vi "whole_setup_control_FPGA_v1229.vi"() -> ()   [LabVIEW 2021]
uses:
  <vilib>/rvi/Emulation/niFpgaSctlEmulationGetInTimedLoop.vi
  <vilib>/rvi/Emulation/niFpgaProcessEmulError.vi
  <vilib>/rvi/Emulation/niFpgaGetClockAttributes.vi
  <vilib>/rvi/Emulation/niFpgaEmulationReportErrorSimple.vi
  <vilib>/rvi/Emulation/niFpgaCriticalErrorInLSC.vi
  <vilib>/rvi/interface/RandomDataEmulation/niFpgaRandomDataHandleErrors.vi
  <vilib>/rvi/Memory/Memory_Emulation/nirvimemoryFastEmulation.vi
  <vilib>/rvi/Memory/Memory_Emulation/nirvimemoryEmulation.vi
  <vilib>/rvi/Emulation/niFpgaEmulationIsFPGAContextNoSignature.vi
  <vilib>/rvi/DataTransferAndStorage/Container/Common/niFpgaContainerGetUniqueNameForEmu.vi
  <vilib>/rvi/errors/nirviReportUnexpectedCaseInternalError (U32).vi
  <vilib>/rvi/eio/common/nirviEmuTemplateMethod_errors.vi
  <vilib>/rvi/DataTransferAndStorage/Container/XNode/niFpgaContainer.xnode
  <vilib>/rvi/interface/RandomDataEmulation/nirviRandomDataFpgaReadWriteTemplate.vi
  <vilib>/eio/EIOMethodNode/EIOMethodNode.xnode
  <vilib>/eio/EIONode/EIONode.xnode
  <vilib>/rvi/FXPMathLib/FxpMul/XNode/nifxpmath_Multiplier.xnode
  <vilib>/rvi/FXPMathLib/FxpAdd/XNode/nifxpmath_Add.xnode
  <vilib>/rvi/FXPMathLib/sim/FxpSim.dll
panel:
  in  "laser ON":bool
  out "Cycle tick spent":u32
  in  "camera trigger ON":bool
  out "FIFO Full? 2":bool
  in  "FPGA loop case":u32 caption="output loop ticks"
  in  "trigger debug?":bool
  in  "DO 4 delay":i32
  in  "DO 3 delay":i32
  in  "camera trigger delay (loops)":i32
  in  "laser delay (loops)":i32
  in  "laser exposure (loops)":i32
  in  "3F0 freq X":i32=3
  in  "2F0 freq X":i32=5
  out "ticks spent update":u32
  out "Loop ticks spent":u32
  in  "Galvo1 offset":fxp<+/-,32,16>
  in  "Galvo1 mag":fxp<+/-,32,16>
  in  "G1 corr amplitude":fxp<+/-,32,16>
  in  "Piezo offset":fxp<+/-,32,16>
  in  "Piezo mag":fxp<+/-,32,16>
  in  "3F0 amplitude":fxp<+/-,32,16>
  in  "2F0 amplitude":fxp<+/-,32,16>
  in  "Galvo1 delay":i32
  in  "Galvo1 corr delay":i32
  in  "stop output":bool
  in  "2F0 phase relative to F0":i32
  in  "3F0 phase relative to F0":i32
  in  "output loop ticks":u32
  in  "output data #":i32
  in  "start output":bool
  in  "array length":i16
  in  "FPGA start to read FIFO":bool
  in  "data row #":i32
  out "Data transfer finished":bool=TRUE
  out "FPGA finish read row":bool
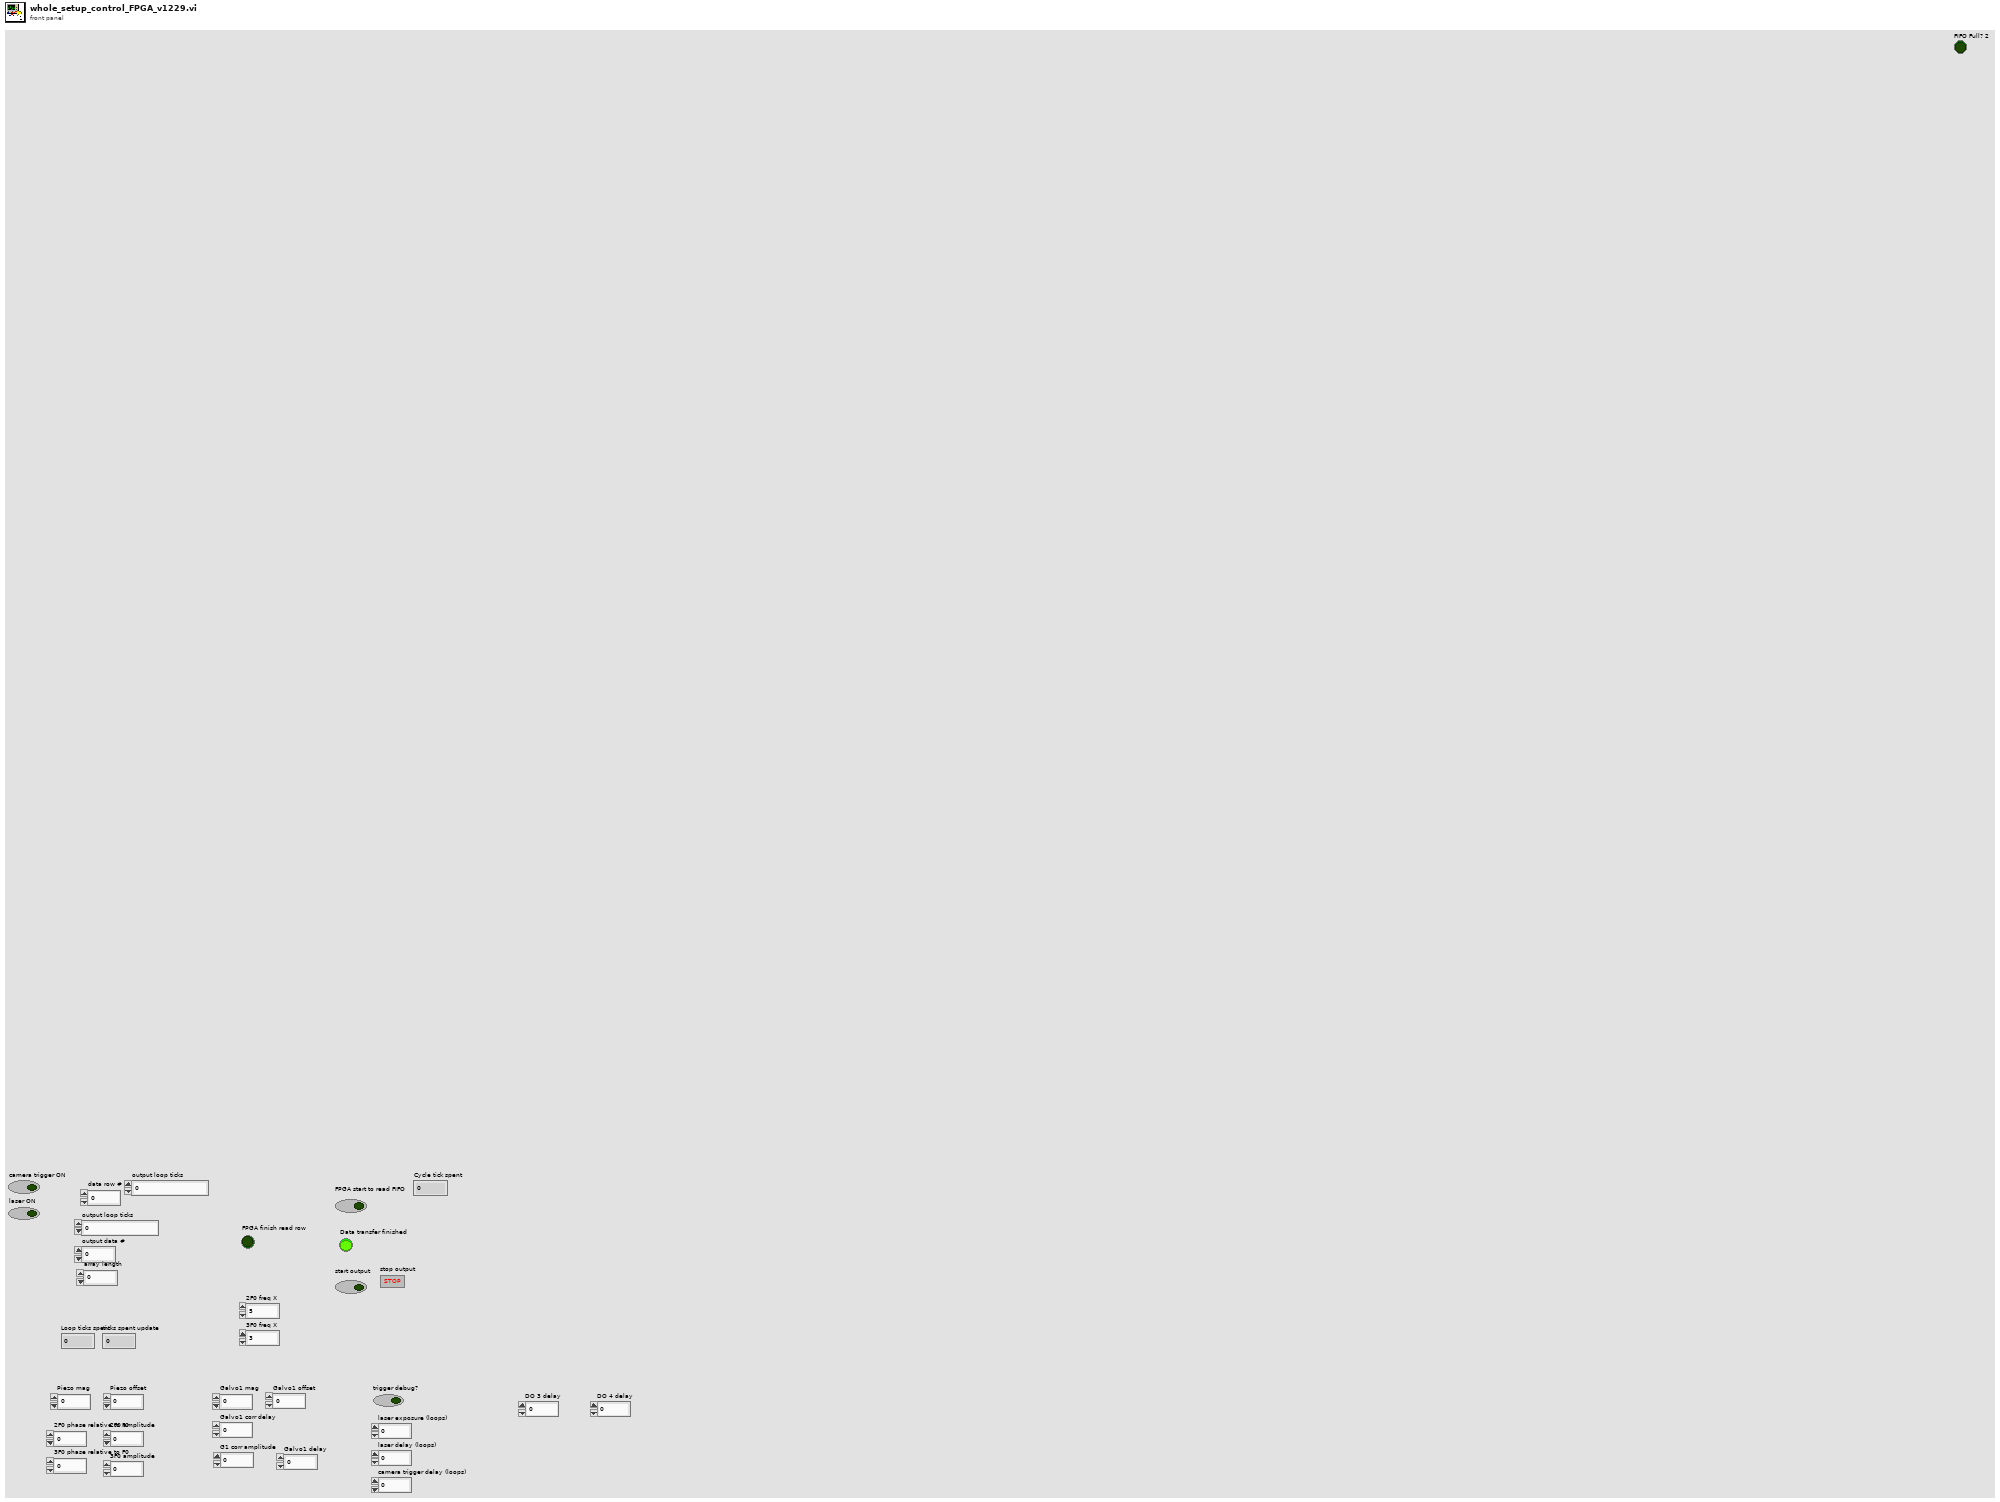
[diagram p1: front panel]
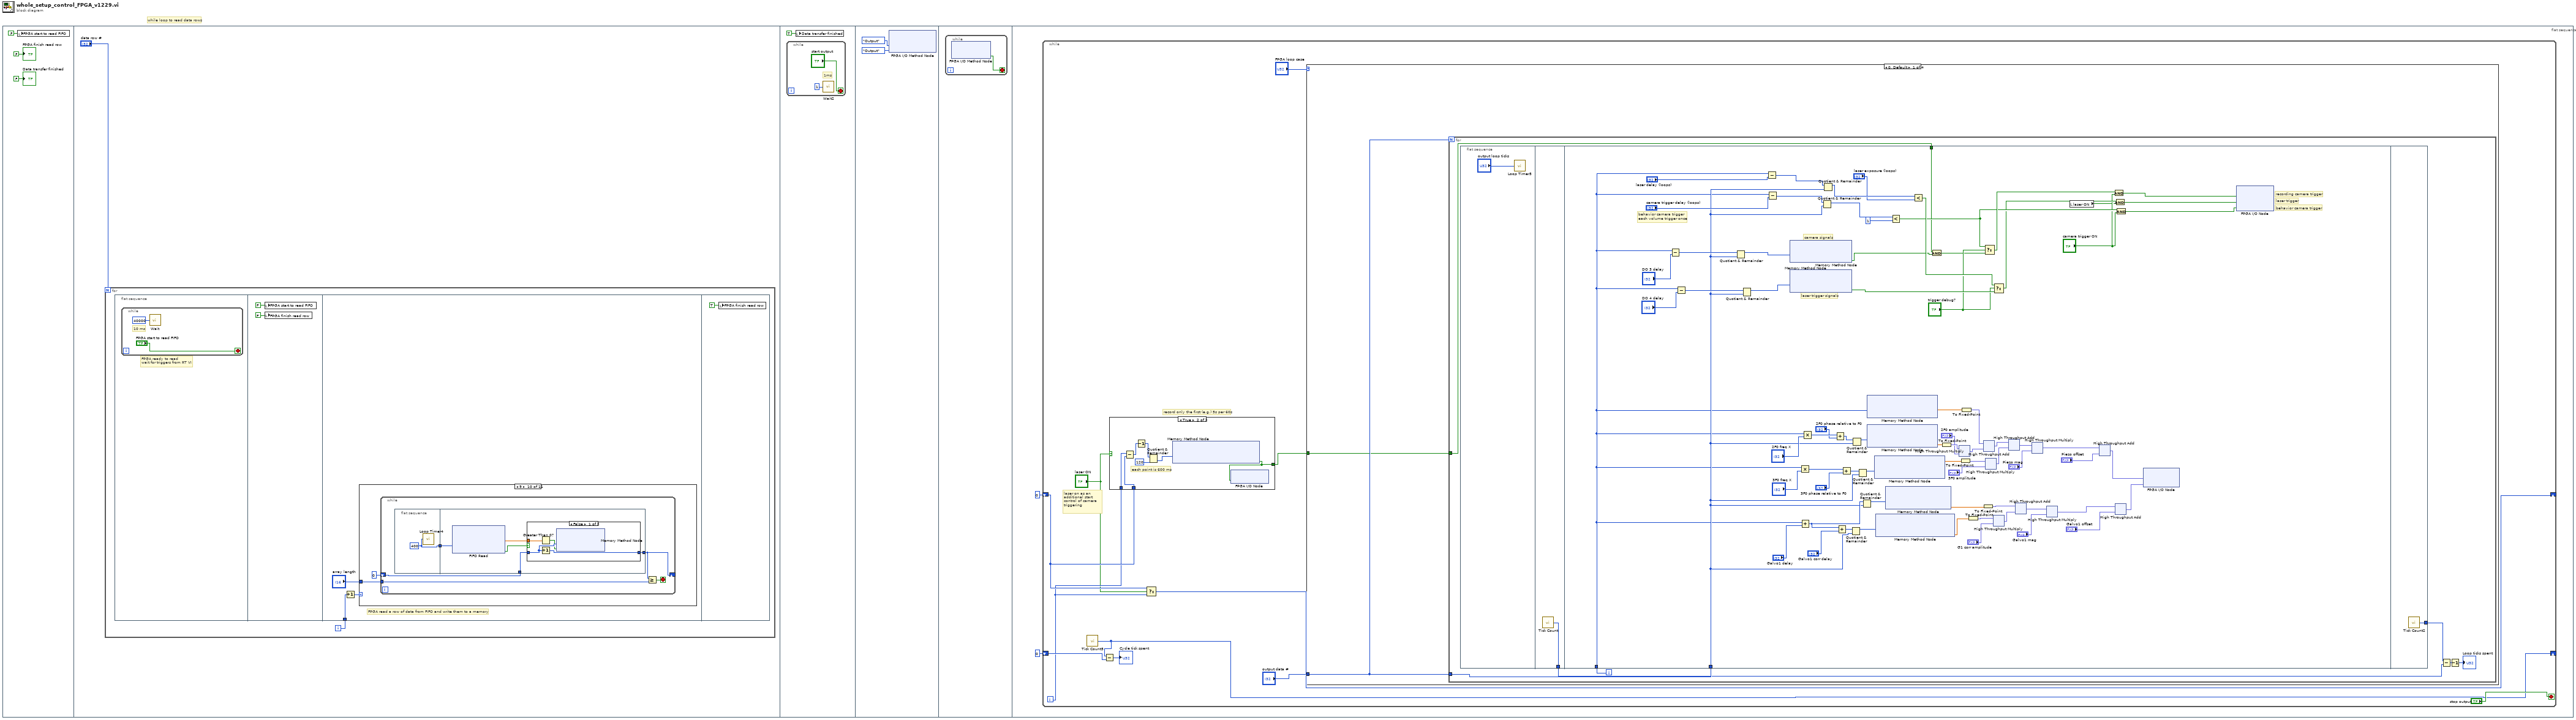
[diagram p0: block diagram]
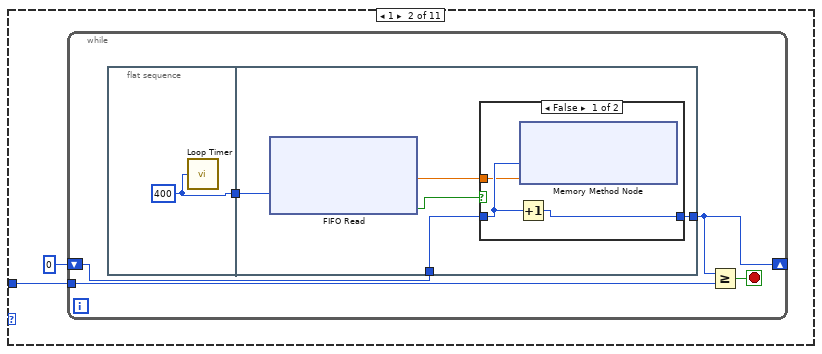
[diagram p3: hidden frame]
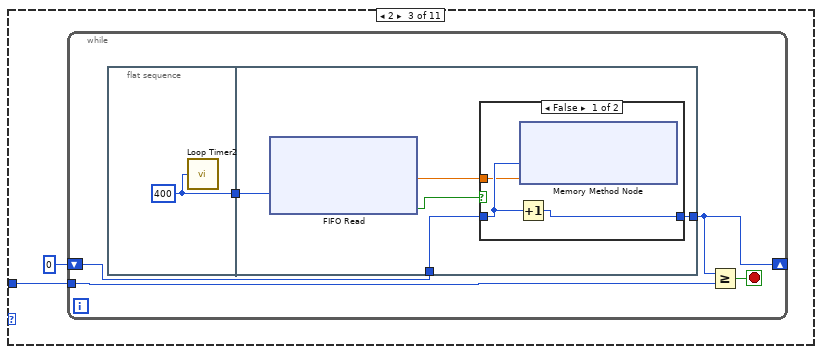
[diagram p5: hidden frame]
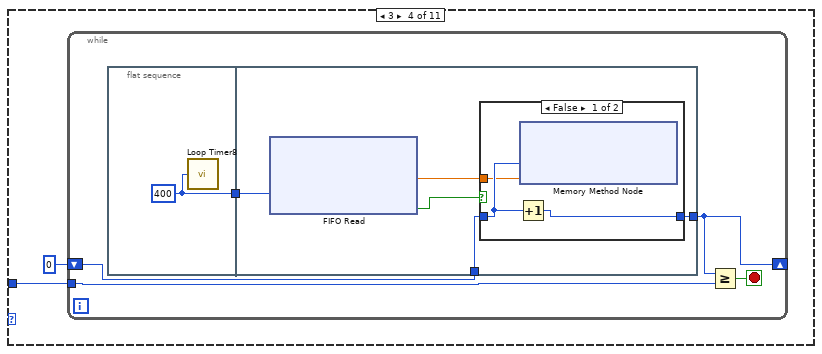
[diagram p7: hidden frame]
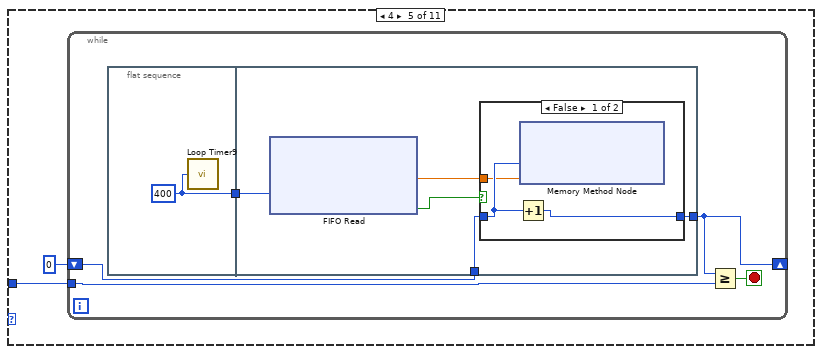
[diagram p9: hidden frame]
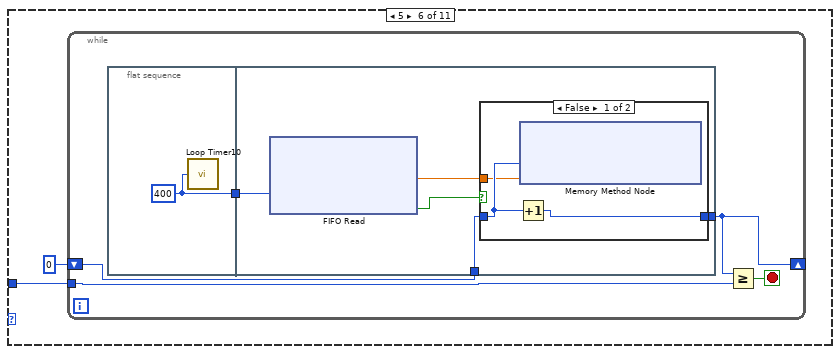
[diagram p11: hidden frame]
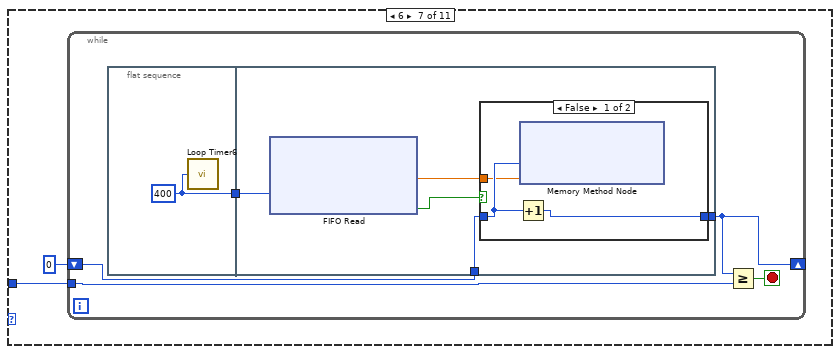
[diagram p13: hidden frame]
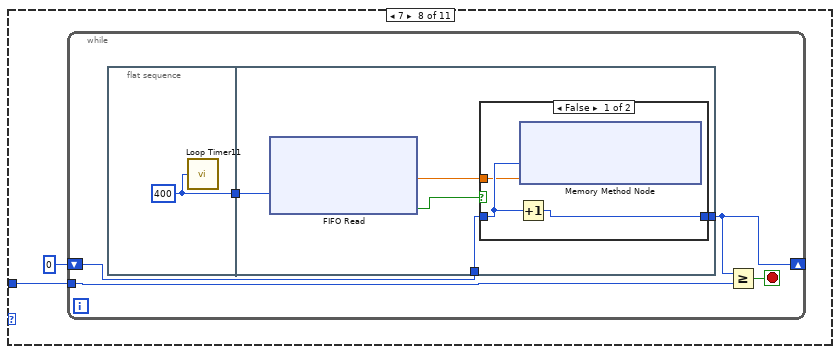
[diagram p15: hidden frame]
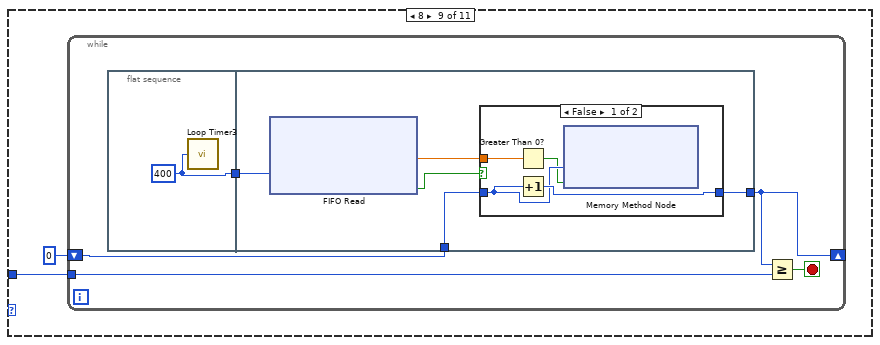
[diagram p17: hidden frame]
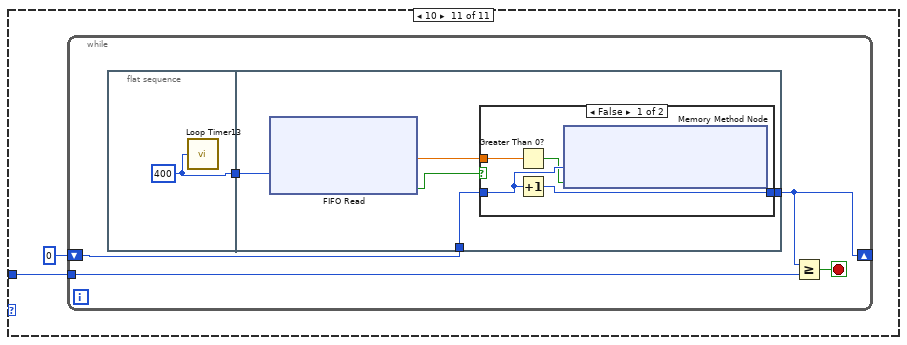
[diagram p20: hidden frame]
diagram:
  # "while loop to read data rows"
  n1 = flat-sequence {
    frame #0 {
      n2 = local write "FPGA start to read FIFO"(FALSE ("FPGA ready to read")) -> ()
      "Data transfer finished" <- FALSE ("Data transfer finished")
      "FPGA finish read row" <- FALSE ("FPGA ready to read")
    }
    frame #1 {
      n3 = for {
        N: "data row #" -> [_]
        i -> [w5]
        n4 = flat-sequence {
          tunnel: w5 -> [w10]
          frame #0 {
            # "FPGA ready to read\nwait for triggers from RT VI"
            n5 = while {
              stop <- "FPGA start to read FIFO" stop-if-true
              # "10 ms"
              n6 = call "Wait"("Count(Ticks)"=u32 40000) -> ()  [unwired: 1 out]
            }
          }
          frame #1 {
            n7 = local write "FPGA start to read FIFO"(FALSE ("FPGA ready to read")) -> ()
            n8 = local write "FPGA finish read row"(FALSE ("FPGA finish read row")) -> ()
          }
          frame #2 {
            # "FPGA read a row of data from FIFO and write them to a memory"
            n9 = Increment(x=w10) -> (x+1=w11:i32)
            n10 = case shown="9" w11 {
              tunnel: "array length" -> [_ w13 w30 w47 w64 w81 w98 w115 w132 w150 w168]
              frame 0, Default {
              }
              frame 1 {
                n11 = while {
                  shift-right: [w15] -> _
                  shift-left: i16 0 -> [w19]
                  tunnel: w13 -> [w16]
                  stop <- w17 stop-if-true
                  n12 = flat-sequence {
                    tunnel: [w20] -> w18
                    tunnel: w19 -> [w24]
                    tunnel: [w23] -> w15
                    tunnel: w18 -> [w21]
                    frame #0 {
                      w20 = u32 400 ("Count(Ticks)")
                      n13 = call "Loop Timer"("Count(Ticks)"=w20) -> ()  [unwired: 1 out]
                    }
                    frame #1 {
                      n14 = xnode ("FIFO Read")("Timeout"=w21) -> ("Element"=w25:sgl, "Timed Out?"=w22:bool)  [unwired: 1 in, 1 out]
                      n15 = case shown="False" w22 {
                        tunnel: w25 -> [w26 _]
                        tunnel: w24 -> [w27 w29]
                        tunnel: [w28 w29] -> w23
                        frame False {
                          n16 = Increment(x=w27) -> (x+1=w28:i16)
                          n17 = xnode ("Memory Method Node")("Address"=w27, "Data"=w26) -> ()  [unwired: 1 in, 1 out]
                        }
                        frame True {
                        }
                      }
                    }
                  }
                  n18 = Greater Or Equal?(x=w15, y=w16) -> (x >= y?=w17:bool)
                }
              }
              frame 2 {
                n19 = while {
                  shift-right: [w32] -> _
                  shift-left: i16 0 -> [w36]
                  tunnel: w30 -> [w33]
                  stop <- w34 stop-if-true
                  n20 = flat-sequence {
                    tunnel: [w37] -> w35
                    tunnel: w36 -> [w41]
                    tunnel: [w40] -> w32
                    tunnel: w35 -> [w38]
                    frame #0 {
                      w37 = u32 400 ("Count(Ticks)")
                      n21 = call "Loop Timer2"("Count(Ticks)"=w37) -> ()  [unwired: 1 out]
                    }
                    frame #1 {
                      n22 = xnode ("FIFO Read")("Timeout"=w38) -> ("Element"=w42:sgl, "Timed Out?"=w39:bool)  [unwired: 1 in, 1 out]
                      n23 = case shown="False" w39 {
                        tunnel: w42 -> [w43 _]
                        tunnel: w41 -> [w44 w46]
                        tunnel: [w45 w46] -> w40
                        frame False {
                          n24 = Increment(x=w44) -> (x+1=w45:i16)
                          n25 = xnode ("Memory Method Node")("Address"=w44, "Data"=w43) -> ()  [unwired: 1 in, 1 out]
                        }
                        frame True {
                        }
                      }
                    }
                  }
                  n26 = Greater Or Equal?(x=w32, y=w33) -> (x >= y?=w34:bool)
                }
              }
              frame 3 {
                n27 = while {
                  shift-right: [w49] -> _
                  shift-left: i16 0 -> [w53]
                  tunnel: w47 -> [w50]
                  stop <- w51 stop-if-true
                  n28 = flat-sequence {
                    tunnel: [w54] -> w52
                    tunnel: w53 -> [w58]
                    tunnel: [w57] -> w49
                    tunnel: w52 -> [w55]
                    frame #0 {
                      w54 = u32 400 ("Count(Ticks)")
                      n29 = call "Loop Timer8"("Count(Ticks)"=w54) -> ()  [unwired: 1 out]
                    }
                    frame #1 {
                      n30 = xnode ("FIFO Read")("Timeout"=w55) -> ("Element"=w59:sgl, "Timed Out?"=w56:bool)  [unwired: 1 in, 1 out]
                      n31 = case shown="False" w56 {
                        tunnel: w59 -> [w60 _]
                        tunnel: w58 -> [w61 w63]
                        tunnel: [w62 w63] -> w57
                        frame False {
                          n32 = Increment(x=w61) -> (x+1=w62:i16)
                          n33 = xnode ("Memory Method Node")("Address"=w61, "Data"=w60) -> ()  [unwired: 1 in, 1 out]
                        }
                        frame True {
                        }
                      }
                    }
                  }
                  n34 = Greater Or Equal?(x=w49, y=w50) -> (x >= y?=w51:bool)
                }
              }
              frame 4 {
                n35 = while {
                  shift-right: [w66] -> _
                  shift-left: i16 0 -> [w70]
                  tunnel: w64 -> [w67]
                  stop <- w68 stop-if-true
                  n36 = flat-sequence {
                    tunnel: [w71] -> w69
                    tunnel: w70 -> [w75]
                    tunnel: [w74] -> w66
                    tunnel: w69 -> [w72]
                    frame #0 {
                      w71 = u32 400 ("Count(Ticks)")
                      n37 = call "Loop Timer9"("Count(Ticks)"=w71) -> ()  [unwired: 1 out]
                    }
                    frame #1 {
                      n38 = xnode ("FIFO Read")("Timeout"=w72) -> ("Element"=w76:sgl, "Timed Out?"=w73:bool)  [unwired: 1 in, 1 out]
                      n39 = case shown="False" w73 {
                        tunnel: w76 -> [w77 _]
                        tunnel: w75 -> [w78 w80]
                        tunnel: [w79 w80] -> w74
                        frame False {
                          n40 = Increment(x=w78) -> (x+1=w79:i16)
                          n41 = xnode ("Memory Method Node")("Address"=w78, "Data"=w77) -> ()  [unwired: 1 in, 1 out]
                        }
                        frame True {
                        }
                      }
                    }
                  }
                  n42 = Greater Or Equal?(x=w66, y=w67) -> (x >= y?=w68:bool)
                }
              }
              frame 5 {
                n43 = while {
                  shift-right: [w83] -> _
                  shift-left: i16 0 -> [w87]
                  tunnel: w81 -> [w84]
                  stop <- w85 stop-if-true
                  n44 = flat-sequence {
                    tunnel: [w88] -> w86
                    tunnel: w87 -> [w92]
                    tunnel: [w91] -> w83
                    tunnel: w86 -> [w89]
                    frame #0 {
                      w88 = u32 400 ("Count(Ticks)")
                      n45 = call "Loop Timer10"("Count(Ticks)"=w88) -> ()  [unwired: 1 out]
                    }
                    frame #1 {
                      n46 = xnode ("FIFO Read")("Timeout"=w89) -> ("Element"=w93:sgl, "Timed Out?"=w90:bool)  [unwired: 1 in, 1 out]
                      n47 = case shown="False" w90 {
                        tunnel: w93 -> [w94 _]
                        tunnel: w92 -> [w95 w97]
                        tunnel: [w96 w97] -> w91
                        frame False {
                          n48 = Increment(x=w95) -> (x+1=w96:i16)
                          n49 = xnode ("Memory Method Node")("Address"=w95, "Data"=w94) -> ()  [unwired: 1 in, 1 out]
                        }
                        frame True {
                        }
                      }
                    }
                  }
                  n50 = Greater Or Equal?(x=w83, y=w84) -> (x >= y?=w85:bool)
                }
              }
              frame 6 {
                n51 = while {
                  shift-right: [w100] -> _
                  shift-left: i16 0 -> [w104]
                  tunnel: w98 -> [w101]
                  stop <- w102 stop-if-true
                  n52 = flat-sequence {
                    tunnel: [w105] -> w103
                    tunnel: w104 -> [w109]
                    tunnel: [w108] -> w100
                    tunnel: w103 -> [w106]
                    frame #0 {
                      w105 = u32 400 ("Count(Ticks)")
                      n53 = call "Loop Timer6"("Count(Ticks)"=w105) -> ()  [unwired: 1 out]
                    }
                    frame #1 {
                      n54 = xnode ("FIFO Read")("Timeout"=w106) -> ("Element"=w110:sgl, "Timed Out?"=w107:bool)  [unwired: 1 in, 1 out]
                      n55 = case shown="False" w107 {
                        tunnel: w110 -> [w111 _]
                        tunnel: w109 -> [w112 w114]
                        tunnel: [w113 w114] -> w108
                        frame False {
                          n56 = Increment(x=w112) -> (x+1=w113:i16)
                          n57 = xnode ("Memory Method Node")("Address"=w112, "Data"=w111) -> ()  [unwired: 1 in, 1 out]
                        }
                        frame True {
                        }
                      }
                    }
                  }
                  n58 = Greater Or Equal?(x=w100, y=w101) -> (x >= y?=w102:bool)
                }
              }
              frame 7 {
                n59 = while {
                  shift-right: [w117] -> _
                  shift-left: i16 0 -> [w121]
                  tunnel: w115 -> [w118]
                  stop <- w119 stop-if-true
                  n60 = flat-sequence {
                    tunnel: [w122] -> w120
                    tunnel: w121 -> [w126]
                    tunnel: [w125] -> w117
                    tunnel: w120 -> [w123]
                    frame #0 {
                      w122 = u32 400 ("Count(Ticks)")
                      n61 = call "Loop Timer11"("Count(Ticks)"=w122) -> ()  [unwired: 1 out]
                    }
                    frame #1 {
                      n62 = xnode ("FIFO Read")("Timeout"=w123) -> ("Element"=w127:sgl, "Timed Out?"=w124:bool)  [unwired: 1 in, 1 out]
                      n63 = case shown="False" w124 {
                        tunnel: w127 -> [w128 _]
                        tunnel: w126 -> [w129 w131]
                        tunnel: [w130 w131] -> w125
                        frame False {
                          n64 = Increment(x=w129) -> (x+1=w130:i16)
                          n65 = xnode ("Memory Method Node")("Address"=w129, "Data"=w128) -> ()  [unwired: 1 in, 1 out]
                        }
                        frame True {
                        }
                      }
                    }
                  }
                  n66 = Greater Or Equal?(x=w117, y=w118) -> (x >= y?=w119:bool)
                }
              }
              frame 8 {
                n67 = while {
                  shift-right: [w134] -> _
                  shift-left: i16 0 -> [w138]
                  tunnel: w132 -> [w135]
                  stop <- w136 stop-if-true
                  n68 = flat-sequence {
                    tunnel: [w139] -> w137
                    tunnel: w138 -> [w143]
                    tunnel: [w142] -> w134
                    tunnel: w137 -> [w140]
                    frame #0 {
                      w139 = u32 400 ("Count(Ticks)")
                      n69 = call "Loop Timer3"("Count(Ticks)"=w139) -> ()  [unwired: 1 out]
                    }
                    frame #1 {
                      n70 = xnode ("FIFO Read")("Timeout"=w140) -> ("Element"=w144:sgl, "Timed Out?"=w141:bool)  [unwired: 1 in, 1 out]
                      n71 = case shown="False" w141 {
                        tunnel: w144 -> [w146 _]
                        tunnel: w143 -> [w147 w149]
                        tunnel: [w148 w149] -> w142
                        frame False {
                          n72 = Greater Than 0?(x=w146) -> (x > 0?=w145:bool)
                          n73 = Increment(x=w147) -> (x+1=w148:i16)
                          n74 = xnode ("Memory Method Node")("Address"=w147, "Data"=w145) -> ()  [unwired: 1 in, 1 out]
                        }
                        frame True {
                        }
                      }
                    }
                  }
                  n75 = Greater Or Equal?(x=w134, y=w135) -> (x >= y?=w136:bool)
                }
              }
              frame 9 {
                n76 = while {
                  shift-right: [w152] -> _
                  shift-left: i16 0 -> [w156]
                  tunnel: w150 -> [w153]
                  stop <- w154 stop-if-true
                  n77 = flat-sequence {
                    tunnel: [w157] -> w155
                    tunnel: w156 -> [w161]
                    tunnel: [w160] -> w152
                    tunnel: w155 -> [w158]
                    frame #0 {
                      w157 = u32 400 ("Count(Ticks)")
                      n78 = call "Loop Timer4"("Count(Ticks)"=w157) -> ()  [unwired: 1 out]
                    }
                    frame #1 {
                      n79 = xnode ("FIFO Read")("Timeout"=w158) -> ("Element"=w162:sgl, "Timed Out?"=w159:bool)  [unwired: 1 in, 1 out]
                      n80 = case shown="False" w159 {
                        tunnel: w162 -> [w164 _]
                        tunnel: w161 -> [w165 w167]
                        tunnel: [w166 w167] -> w160
                        frame False {
                          n81 = Greater Than 0?(x=w164) -> (x > 0?=w163:bool)
                          n82 = Increment(x=w165) -> (x+1=w166:i16)
                          n83 = xnode ("Memory Method Node")("Address"=w165, "Data"=w163) -> ()  [unwired: 1 in, 1 out]
                        }
                        frame True {
                        }
                      }
                    }
                  }
                  n84 = Greater Or Equal?(x=w152, y=w153) -> (x >= y?=w154:bool)
                }
              }
              frame 10 {
                n85 = while {
                  shift-right: [w170] -> _
                  shift-left: i16 0 -> [w174]
                  tunnel: w168 -> [w171]
                  stop <- w172 stop-if-true
                  n86 = flat-sequence {
                    tunnel: [w175] -> w173
                    tunnel: w174 -> [w179]
                    tunnel: [w178] -> w170
                    tunnel: w173 -> [w176]
                    frame #0 {
                      w175 = u32 400 ("Count(Ticks)")
                      n87 = call "Loop Timer13"("Count(Ticks)"=w175) -> ()  [unwired: 1 out]
                    }
                    frame #1 {
                      n88 = xnode ("FIFO Read")("Timeout"=w176) -> ("Element"=w180:sgl, "Timed Out?"=w177:bool)  [unwired: 1 in, 1 out]
                      n89 = case shown="False" w177 {
                        tunnel: w180 -> [w182 _]
                        tunnel: w179 -> [w183 w185]
                        tunnel: [w184 w185] -> w178
                        frame False {
                          n90 = Greater Than 0?(x=w182) -> (x > 0?=w181:bool)
                          n91 = Increment(x=w183) -> (x+1=w184:i16)
                          n92 = xnode ("Memory Method Node")("Address"=w183, "Data"=w181) -> ()  [unwired: 1 in, 1 out]
                        }
                        frame True {
                        }
                      }
                    }
                  }
                  n93 = Greater Or Equal?(x=w170, y=w171) -> (x >= y?=w172:bool)
                }
              }
            }
          }
          frame #3 {
            n94 = local write "FPGA finish read row"(TRUE ("FPGA finish read row")) -> ()
          }
        }
      }
    }
    frame #2 {
      n95 = while {
        stop <- "start output" stop-if-true
        # "1ms"
        n96 = call "Wait2"("Count(mSec)"=u32 1) -> ()  [unwired: 1 out]
      }
      n97 = local write "Data transfer finished"(TRUE ("Data transfer finished")) -> ()
    }
    frame #3 {
      n98 = xnode "FPGA I/O Method Node"("DIO 7:4"=enum8{"No Change", "Input", "Output"}."Output", "DIO 3:0"=enum8{"No Change", "Input", "Output"}."Output") -> ()  [unwired: 1 in, 1 out]
    }
    frame #4 {
      n99 = while {
        stop <- w192 stop-if-true
        n100 = xnode "FPGA I/O Method Node"() -> ("Ready"=w192:bool)  [unwired: 2 in, 2 out]
      }
    }
    frame #5 {
      n101 = while {
        shift-right: [w202] -> _
        shift-left: u32 0 ("Tick Count(Ticks)") -> [w201]
        shift-right: [w199] -> _
        shift-left: 0 -> [w198]
        i -> [w197]
        stop <- "stop output" stop-if-true
        # "record only the first (e.g.) 5s per 60s"
        # "laser on as an additional start control of camera triggering"
        n102 = call "Tick Count5"() -> ("Tick Count(Ticks)"=w202:u32)
        n103 = Subtract(x=w202, y=w201) -> (x-y=→"Cycle tick spent":u32)
        n104 = case shown="True" "laser ON" {
          tunnel: w198 -> [_ w213]
          tunnel: w197 -> [_ w212]
          tunnel: [w206 w207] -> w195
          frame False {
            w206 = FALSE ("Mod1/DIO3")
            n105 = xnode "FPGA I/O Node"("Mod1/DIO3"=w206) -> ()  [unwired: 1 in, 1 out]
          }
          frame True {
            # "each point is 600 ms"
            n106 = Subtract(x=w212, y=w213) -> (x-y=w209:i32)
            n107 = Decrement(x=w209) -> (x-1=w208:i32)
            n108 = Quotient & Remainder(x=w208, y=120) -> (floor(x/y)=w211:i32)  [unwired: 1 out]
            n109 = xnode ("Memory Method Node")("Address"=w211) -> ("Data"=w207:bool)  [unwired: 1 in, 1 out]
            n110 = xnode "FPGA I/O Node"("Mod1/DIO3"=w207) -> ()  [unwired: 1 in, 1 out]
          }
        }
        n111 = Select(t=w198, s="laser ON", f=w197) -> (s? t:f=w199:i32)
        n112 = case shown="0, Default" "FPGA loop case" {
          tunnel: "output data #" -> [w215 w300 w326 _]
          tunnel: w195 -> [w214 _ _ _]
          frame 0, Default {
            n113 = for {
              N: w215 -> [_]
              tunnel: w215 -> [w221]
              tunnel: w214 -> [w216]
              i -> [w222]
              n114 = flat-sequence {
                tunnel: [w224] -> w218
                tunnel: w222 -> [w237]
                tunnel: w221 -> [w238]
                tunnel: w216 -> [w229]
                tunnel: [w298] -> w217
                frame #0 {
                  n115 = call "Loop Timer5"("Count(Ticks)"="output loop ticks") -> ()  [unwired: 1 out]
                }
                frame #1 {
                  n116 = call "Tick Count"() -> ("Tick Count(Ticks)"=w224:u32)
                }
                frame #2 {
                  # "recording camera trigger"
                  # "laser trigger"
                  # "behavior camera trigger"
                  # "behavior camera trigger\neach volume trigger once"
                  # "laser trigger signals"
                  # "camera signals"
                  n117 = Subtract(x=w237, y="DO 3 delay") -> (x-y=w248:i32)
                  n118 = Subtract(x=w237, y="DO 4 delay") -> (x-y=w245:i32)
                  n119 = Quotient & Remainder(x=w248, y=w238) -> (x-y*floor(x/y)=w247:i32)  [unwired: 1 out]
                  n120 = Quotient & Remainder(x=w245, y=w238) -> (x-y*floor(x/y)=w243:i32)  [unwired: 1 out]
                  n121 = Subtract(x=w237, y="laser delay (loops)") -> (x-y=w252:i32)
                  n122 = Subtract(x=w237, y="camera trigger delay (loops)") -> (x-y=w250:i32)
                  n123 = xnode ("Memory Method Node")("Address"=w247) -> ("Data"=w228:bool)  [unwired: 1 in, 1 out]
                  n124 = xnode ("Memory Method Node")("Address"=w243) -> ("Data"=w242:bool)  [unwired: 1 in, 1 out]
                  n125 = Multiply(x=w237, y="3F0 freq X") -> (x*y=w297:i32)
                  n126 = Add(x=w237, y="Galvo1 delay") -> (x+y=w258:i32)
                  n127 = Multiply(x=w237, y="2F0 freq X") -> (x*y=w293:i32)
                  n128 = Quotient & Remainder(x=w250, y=w238) -> (x-y*floor(x/y)=w225:i32)  [unwired: 1 out]
                  n129 = Quotient & Remainder(x=w252, y=w238) -> (x-y*floor(x/y)=w254:i32)  [unwired: 1 out]
                  n130 = Add(x=w293, y="2F0 phase relative to F0") -> (x+y=w296:i32)
                  n131 = Add(x=w258, y="Galvo1 corr delay") -> (x+y=w286:i32)
                  n132 = Add(x=w297, y="3F0 phase relative to F0") -> (x+y=w290:i32)
                  n133 = Quotient & Remainder(x=w286, y=w238) -> (x-y*floor(x/y)=w288:i32)  [unwired: 1 out]
                  n134 = Quotient & Remainder(x=w296, y=w238) -> (x-y*floor(x/y)=w295:i32)  [unwired: 1 out]
                  n135 = Quotient & Remainder(x=w290, y=w238) -> (x-y*floor(x/y)=w289:i32)  [unwired: 1 out]
                  n136 = Quotient & Remainder(x=w258, y=w238) -> (x-y*floor(x/y)=w256:i32)  [unwired: 1 out]
                  n137 = xnode ("Memory Method Node")("Address"=w237) -> ("Data"=w284:sgl)  [unwired: 1 in, 1 out]
                  n138 = xnode ("Memory Method Node")("Address"=w295) -> ("Data"=w279:sgl)  [unwired: 1 in, 1 out]
                  n139 = xnode ("Memory Method Node")("Address"=w289) -> ("Data"=w280:sgl)  [unwired: 1 in, 1 out]
                  n140 = xnode ("Memory Method Node")("Address"=w288) -> ("Data"=w282:sgl)  [unwired: 1 in, 1 out]
                  n141 = xnode ("Memory Method Node")("Address"=w256) -> ("Data"=w281:sgl)  [unwired: 1 in, 1 out]
                  n142 = Less?(x=w225, y=1) -> (x < y?=w236:bool)
                  n143 = Less?(x=w254, y="laser exposure (loops)") -> (x < y?=w239:bool)
                  n144 = And(x=w229, y=w228) -> (x .and. y?=w227:bool)
                  n145 = To Fixed-Point(number=w279) -> (fixed-point=w278:fxp<+/-,32,16>)  [unwired: 1 in]
                  n146 = xnode ("High Throughput Multiply")("x"=w278, "y"="2F0 amplitude") -> ("x*y"=w277:fxp<+/-,32,16>)
                  n147 = To Fixed-Point(number=w280) -> (fixed-point=w274:fxp<+/-,32,16>)  [unwired: 1 in]
                  n148 = To Fixed-Point(number=w284) -> (fixed-point=w283:fxp<+/-,32,16>)  [unwired: 1 in]
                  n149 = To Fixed-Point(number=w282) -> (fixed-point=w260:fxp<+/-,32,16>)  [unwired: 1 in]
                  n150 = To Fixed-Point(number=w281) -> (fixed-point=w261:fxp<+/-,32,16>)  [unwired: 1 in]
                  n151 = xnode ("High Throughput Add")("x"=w283, "y"=w277) -> ("x+y"=w275:fxp<+/-,32,16>)
                  n152 = Select(t=w236, s="trigger debug?", f=w227) -> (s? t:f=w241:bool)
                  n153 = xnode ("High Throughput Multiply")("x"=w274, "y"="3F0 amplitude") -> ("x*y"=w272:fxp<+/-,32,16>)
                  n154 = Select(t=w239, s="trigger debug?", f=w242) -> (s? t:f=w233:bool)
                  n155 = xnode ("High Throughput Multiply")("x"=w260, "y"="G1 corr amplitude") -> ("x*y"=w266:fxp<+/-,32,16>)
                  n156 = xnode ("High Throughput Add")("x"=w275, "y"=w272) -> ("x+y"=w271:fxp<+/-,32,16>)
                  n157 = xnode ("High Throughput Add")("x"=w261, "y"=w266) -> ("x+y"=w257:fxp<+/-,32,16>)
                  n158 = xnode ("High Throughput Multiply")("x"=w271, "y"="Piezo mag") -> ("x*y"=w269:fxp<+/-,32,16>)
                  n159 = xnode ("High Throughput Multiply")("x"=w257, "y"="Galvo1 mag") -> ("x*y"=w263:fxp<+/-,32,16>)
                  n160 = local read "laser ON"() -> (w230:bool)
                  n161 = xnode ("High Throughput Add")("x"=w269, "y"="Piezo offset") -> ("x+y"=w267:fxp<+/-,32,16>)
                  n162 = And(x=w241, y="camera trigger ON") -> (x .and. y?=w226:bool)
                  n163 = And(x=w233, y=w230) -> (x .and. y?=w232:bool)
                  n164 = xnode ("High Throughput Add")("x"=w263, "y"="Galvo1 offset") -> ("x+y"=w259:fxp<+/-,32,16>)
                  n165 = And(x=w236, y="camera trigger ON") -> (x .and. y?=w235:bool)
                  n166 = xnode "FPGA I/O Node"("Mod2/AO0"=w267, "Mod2/AO1"=w259) -> ()  [unwired: 2 in, 2 out]
                  n167 = xnode "FPGA I/O Node"("Mod1/DIO0"=w226, "Mod1/DIO1"=w232, "Mod1/DIO2"=w235) -> ()  [unwired: 3 in, 3 out]
                }
                frame #3 {
                  n168 = call "Tick Count2"() -> ("Tick Count(Ticks)"=w298:u32)
                }
              }
              n169 = Subtract(x=w217, y=w218) -> (x-y=w220:u32)
              n170 = Decrement(x=w220) -> (x-1=→"Loop ticks spent":u32)
            }
          }
          frame 1 {
            n171 = for {
              N: w300 -> [_]
              tunnel: w300 -> [w301]
              i -> [w306]
              n172 = flat-sequence {
                tunnel: [w308] -> w303
                tunnel: w306 -> [w310]
                tunnel: w301 -> [w309]
                tunnel: [w325] -> w302
                frame #0 {
                  n173 = call "Loop Timer7"("Count(Ticks)"=u32 400) -> ()  [unwired: 1 out]
                }
                frame #1 {
                  n174 = call "Tick Count3"() -> ("Tick Count(Ticks)"=w308:u32)
                }
                frame #2 {
                  n175 = local read "Galvo1 delay"() -> (w313:i32)
                  n176 = local read "Galvo1 corr delay"() -> (w312:i32)
                  n177 = Add(x=w310, y=w313) -> (x+y=w317:i32)
                  n178 = Add(x=w317, y=w312) -> (x+y=w323:i32)
                  n179 = Quotient & Remainder(x=w323, y=w309) -> (x-y*floor(x/y)=w324:i32)  [unwired: 1 out]
                  n180 = Quotient & Remainder(x=w317, y=w309) -> (x-y*floor(x/y)=w314:i32)  [unwired: 1 out]
                  n181 = xnode ("Memory Method Node")("Address"=w324) -> ("Data"=w322:sgl)  [unwired: 1 in, 1 out]
                  n182 = xnode ("Memory Method Node")("Address"=w314) -> ("Data"=w321:sgl)  [unwired: 1 in, 1 out]
                  n183 = local read "G1 corr amplitude"() -> (w311:fxp<+/-,32,16>)
                  n184 = To Fixed-Point(number=w321) -> (fixed-point=w319:fxp<+/-,32,16>)  [unwired: 1 in]
                  n185 = To Fixed-Point(number=w322) -> (fixed-point=w318:fxp<+/-,32,16>)  [unwired: 1 in]
                  n186 = xnode ("High Throughput Multiply")("x"=w318, "y"=w311) -> ("x*y"=w320:fxp<+/-,32,16>)
                  n187 = xnode ("High Throughput Add")("x"=w319, "y"=w320) -> ("x+y"=w315:fxp<+/-,32,16>)
                  n188 = To Single Precision Float(number=w315) -> (single precision float=w316:sgl)
                  n189 = xnode ("Memory Write")("Address"=w314, "Data"=w316) -> ()  [unwired: 1 in, 1 out]
                }
                frame #3 {
                  n190 = call "Tick Count4"() -> ("Tick Count(Ticks)"=w325:u32)
                }
              }
              n191 = Subtract(x=w302, y=w303) -> (x-y=w305:u32)
              n192 = Decrement(x=w305) -> (x-1=→"ticks spent update":u32)
            }
            n193 = local write "FPGA loop case"(u32 0 ("FPGA loop case")) -> ()
          }
          frame 2 {
            n194 = for {
              N: w326 -> [_]
              i -> [w330]
              n195 = flat-sequence {
                tunnel: [w331] -> w329
                tunnel: w330 -> [w335]
                tunnel: w329 -> [w333]
                tunnel: [w332] -> w328
                frame #0 {
                  w331 = u32 400 ("Count(Ticks)")
                  n196 = call "Loop Timer12"("Count(Ticks)"=w331) -> ()  [unwired: 1 out]
                }
                frame #1 {
                  n197 = xnode ("Memory Method Node")("Address"=w335) -> ("Data"=w334:sgl)  [unwired: 1 in, 1 out]
                  n198 = xnode ("FIFO Method Node")("Element"=w334, "Timeout"=w333) -> ("Timed Out?"=w332:bool)  [unwired: 1 in, 1 out]
                }
              }
              "FIFO Full? 2" <- w328
            }
            n199 = local write "FPGA loop case"(u32 0 ("FPGA loop case")) -> ()
          }
          frame 3 {
            n200 = local read "array length"() -> (w336:i16)
            n201 = while {
              shift-right: [w339] -> _
              shift-left: i16 0 -> [w343]
              tunnel: w336 -> [w340]
              stop <- w341 stop-if-true
              n202 = flat-sequence {
                tunnel: [w344] -> w342
                tunnel: w343 -> [w348]
                tunnel: [w347] -> w339
                tunnel: w342 -> [w345]
                frame #0 {
                  w344 = u32 400 ("Count(Ticks)")
                  n203 = call "Loop Timer14"("Count(Ticks)"=w344) -> ()  [unwired: 1 out]
                }
                frame #1 {
                  n204 = xnode ("FIFO Read")("Timeout"=w345) -> ("Element"=w349:sgl, "Timed Out?"=w346:bool)  [unwired: 1 in, 1 out]
                  n205 = case shown="False" w346 {
                    tunnel: w349 -> [w352 _]
                    tunnel: w348 -> [w351 w354]
                    tunnel: [w353 w354] -> w347
                    frame False {
                      n206 = Greater Than 0?(x=w352) -> (x > 0?=w350:bool)
                      n207 = Increment(x=w351) -> (x+1=w353:i16)
                      n208 = xnode ("Memory Method Node")("Address"=w351, "Data"=w350) -> ()  [unwired: 1 in, 1 out]
                      n209 = xnode ("Memory Method Node")("Address"=w351, "Data"=w350) -> ()  [unwired: 1 in, 1 out]
                    }
                    frame True {
                    }
                  }
                }
              }
              n210 = Greater Or Equal?(x=w339, y=w340) -> (x >= y?=w341:bool)
            }
            n211 = local write "FPGA loop case"(u32 0 ("FPGA loop case")) -> ()
          }
        }
      }
    }
  }
